vi "ELVIS III v1.0 RPC Unreserve Resouce.vi"(7 "Allow multiple opens?":bool, 8 "error in (no error)":errorcluster, 10 "Channel Reservation List":T1, 11 "Owner":string) -> (0 "error out":errorcluster, 3 "Session":u32)   [LabVIEW 2021]
uses:
  <vilib>/myRIO/Common/Instrument Driver Framework/ELVIS III v1.0/Resource Manager/typedefs/ELVIS III v1.0 Channel Reservation List.ctl
  <vilib>/myRIO/Common/Instrument Driver Framework/ELVIS III v1.0/Resource Manager/typedefs/ELVIS III v1.0 Channel Reservation Info.ctl
  <vilib>/myRIO/Common/Instrument Driver Framework/ELVIS III v1.0/Resource Manager/typedefs/ELVIS III v1.0 Connector List.ctl
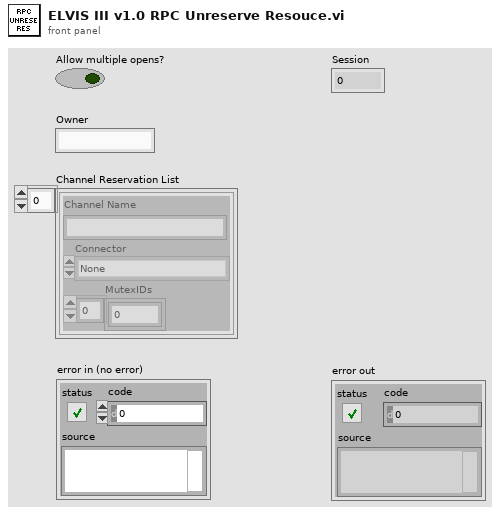
[diagram p1: front panel]
types:
  T1 = typedef "ELVIS III v1.0 Channel Reservation List.ctl" = T2[]
  T2 = typedef "ELVIS III v1.0 Channel Reservation Info.ctl" = cluster{"Channel Name":string, "Connector":T3, "MutexIDs":u32[]}
  T3 = typedef "ELVIS III v1.0 Connector List.ctl" = enum32{"None", "ConnectorA", "ConnectorB"}
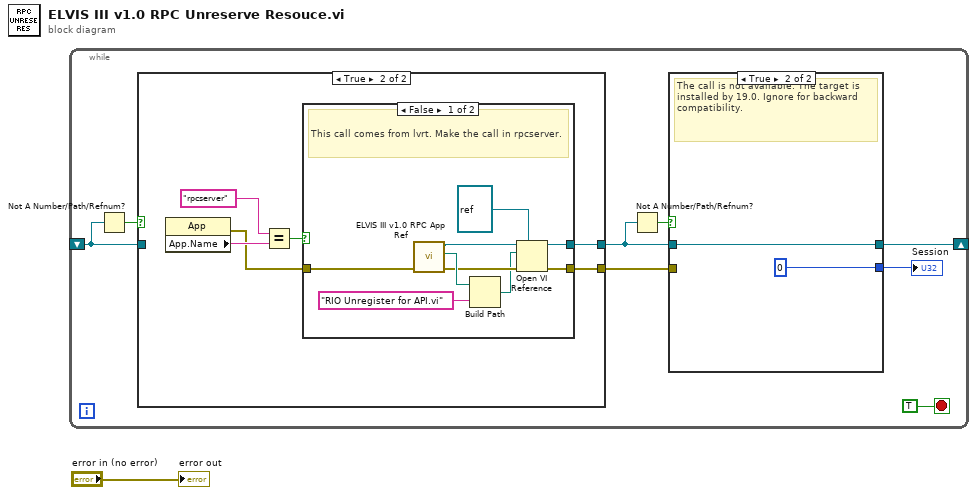
[diagram p0: block diagram]
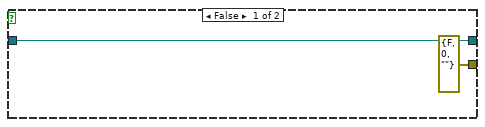
[diagram p2: hidden frame]
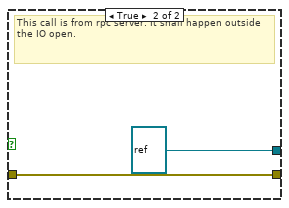
[diagram p3: hidden frame]
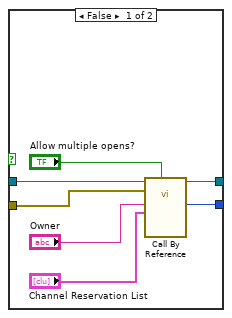
[diagram p4: hidden frame]
diagram:
  n1 = while {
    shift-right: [w6] -> _
    shift-left: _ -> [w4]
    stop <- TRUE stop-if-true
    n2 = Not A Number/Path/Refnum?(number/path/refnum=w4) -> (NaN/Path/Refnum?=w5:bool)
    n3 = case shown="True" w5 {
      tunnel: [w11 w14] -> w8
      tunnel: w4 -> [w11 _]
      tunnel: [errorcluster {"status"=FALSE, "code"=0, "source"=""} ("error out") w12] -> w3
      frame False {
      }
      frame True {
        n4 = property class="App"() -> (error out=w13:errorcluster, "App.Name"=w17:string)  [unwired: 2 in, 1 out]
        n5 = Equal?(x="rpcserver" ("Application:Name"), y=w17) -> (x = y?=w16:bool)
        n6 = case shown="False" w16 {
          tunnel: [w24 refnum<vi> refnum ("type specifier VI Refnum (for type only)")] -> w14
          tunnel: w13 -> [w19 w26]
          tunnel: [w23 w26] -> w12
          frame False {
            # "This call comes from lvrt. Make the call in rpcserver."
            n7 = call <vilib>:"ELVIS III v1.0 RPC App Ref.vi"() -> ("Lib Path"=w22:path, "RPC Reference"=w20:refnum<vi>)  [unwired: 10 in]
            n8 = Build Path(base path=w22, name or relative path="RIO Unregister for API.vi") -> (appended path=w18:path)
            n9 = Open VI Reference(type specifier VI Refnum (for type only)=refnum<vi> refnum, application reference (local)=w20, vi path=w18, error in (no error)=w19) -> (vi reference=w24:refnum<vi>, error out=w23:errorcluster)  [unwired: 2 in]
          }
          frame True {
            # "This call is from rpc server. It shall happen outside the IO open."
          }
        }
      }
    }
    n10 = Not A Number/Path/Refnum?(number/path/refnum=w8) -> (NaN/Path/Refnum?=w9:bool)
    n11 = case shown="True" w9 {
      tunnel: w8 -> [w34 w36]
      tunnel: [w33 w36] -> w6
      tunnel: w3 -> [w32 _]
      tunnel: [w28 u32 0 ("Session")] -> w2
      frame False {
        n12 = call-by-ref "?"(reference=w34, error in=w32, "Allow multiple opens?"="Allow multiple opens?", "Channel Reservation List"="Channel Reservation List", "Owner"="Owner") -> (reference out=w33:refnum<vi>, "Session"=w28:u32)  [unwired: 7 in, 2 out]
      }
      frame True {
        # "The call is not available. The target is installed by 19.0. Ignore for backward compatibility."
      }
    }
    "Session" <- w2
  }
  "error out" <- "error in (no error)"
